vi "Accumulate Gyro.vi"(1 "Gyro Rate":dbl) -> (0 "Accumulated Gyro":dbl)   [LabVIEW 2014]
panel:
  in  "Dividing by":u32
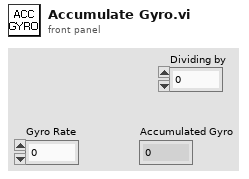
[diagram p1: front panel]
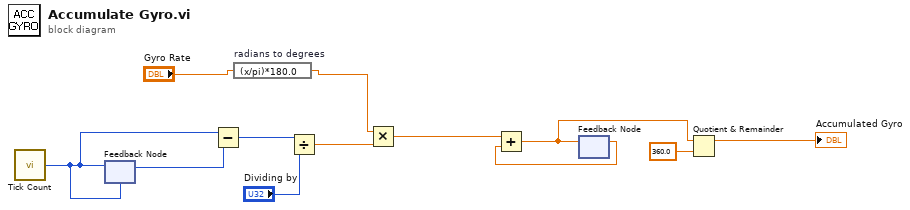
[diagram p0: block diagram]
diagram:
  n1 = call "Tick Count"() -> ("Tick Count(mSec)"=w12:u32)
  n2 = feedback-in #1(w12) -> ()
  n3 = feedback #1(w12) -> (w11:u32)
  n4 = Subtract(x=w12, y=w11) -> (x-y=w5:u32)
  n5 = expression code="(x/pi)*180.0" "radians to degrees"("Gyro Rate") -> (w2:dbl)
  n6 = Divide(x=w5, y="Dividing by") -> (x/y=w3:dbl)
  n7 = Multiply(x=w2, y=w3) -> (x*y=w10:dbl)
  n8 = feedback #2() -> (w9:dbl)  [unwired: 1 in]
  n9 = Add(x=w10, y=w9) -> (x+y=w8:dbl)
  n10 = feedback-in #2(w8) -> ()
  n11 = Quotient & Remainder(x=w8, y=360.0) -> (x-y*floor(x/y)=→"Accumulated Gyro":dbl)  [unwired: 1 out]
